vi "Send Command.vi"(6 "Command in":T1, 8 "error in (no error)":errorcluster, 10 "Value":dbl, 11 "Hitronics in":refnum<class "Hitronics.lvclass">) -> (0 "error out":errorcluster, 3 "Hitronics out":refnum<class "Hitronics.lvclass">, 4 "Command out":T1)   [LabVIEW 2018, in "Hitronics.lvlib" / "Hitronics.lvclass"]
doc: "Send commands to laser."
uses:
  Hitronics.lvclass
  PPLs/Laser/Parent/Laser.lvlibp/Custom Controls/Command List.ctl
  PPLs/Laser/Parent/Laser.lvlibp/Laser.lvclass
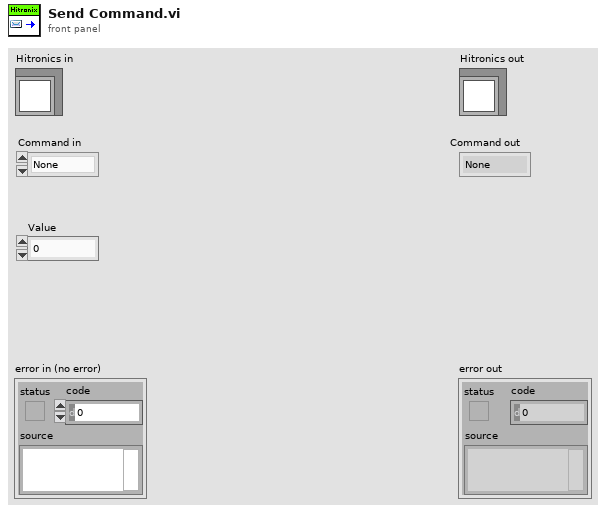
[diagram p1: front panel]
types:
  T1 = typedef "Laser.lvlibp/Laser.lvclass/Command List.ctl" = enum16{"None", "Config?", "Volt?", "ThCase?", "STS?", "Mon?", "Help?", "HB", "Verbose", "Spnt", "Ext", "PRF", "Start", "Stop", "PRF?", "State?", "Status?", "Stat?", "Read HB", "Logon", "Poutmax", "saveconfig", "Reset", "Poutmax?", "PoutCommandMax", "PoutCommandMax?", "FreqMin", "FreqMin?"}
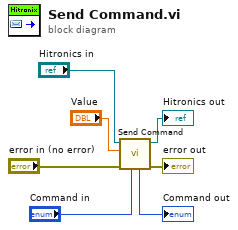
[diagram p0: block diagram]
diagram:
  n1 = call-parent "Send Command.vi"("Command in"="Command in", "error in (no error)"="error in (no error)", "Value"="Value", "Laser in"="Hitronics in") -> ("error out"=→"error out":errorcluster, "Laser out"=→"Hitronics out":refnum<class "Hitronics.lvclass">, "Command out"=→"Command out":T1)  [unwired: 5 in]
